vi "DWF Dig Query Line Configuration.vi"(0 "Instrument Handle In":u32, 11 "Error In":errorcluster caption="Error In (no error)") -> (4 "Instrument Handle Out":u32, 6 "Tristate Lines":string caption="Trigger Pattern", 8 "Static Lines":string caption="Trigger Pattern", 15 "Error Out":errorcluster)   [LabVIEW 2015, in "DigilentWF.lvlib"]
doc: "Indicates the current line configurations. <B>Tristate Lines</B>, <B>Static Lines</B>, and <B>Export Lines</B> contain comma-separated range and/or colon-delimited lists of all lines specified in Dig Initialize"
uses:
  <vilib>/DigilentWF/DigilentWF.lvlib
  dwf.dll
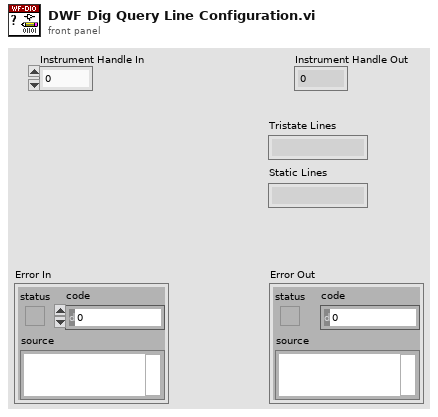
[diagram p1: front panel]
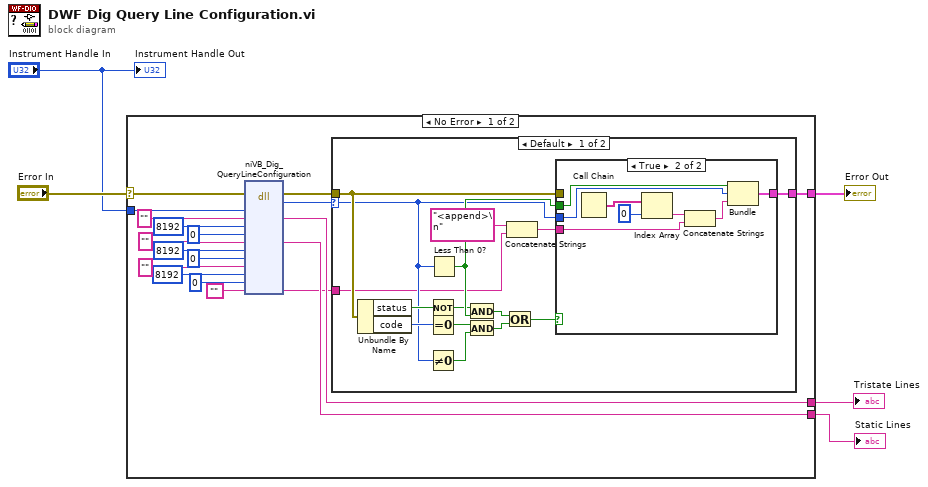
[diagram p0: block diagram]
diagram:
  n1 = case "outter_case" shown="No Error" "Error In" {
    selector: "Error In" -> [w19 w49]
    tunnel: [w23 w49] -> w4
    tunnel: "Instrument Handle In" -> [w10 _]
    tunnel: [w9 _] -> w2
    tunnel: [w8 _] -> w1
    frame No Error {
      n2 = dll-call lib="dwf.*" fn="niVB_Dig_QueryLineConfiguration"(error in=w19, "instrumentHandle"=w10, "tristateLines"="", "tristateLinesSize"=8192, "tristateLinesSizeOut"=0, "staticLines"="", "staticLinesSize"=8192, "staticLinesSizeOut"=0, "exportLines"="", "exportLinesSize"=8192, "exportLinesSizeOut"=0, "szError"="") -> (error out=w18:errorcluster, "return type"=w11:u32, "tristateLines"=w9:string, "staticLines"=w8:string, "szError"=w6:string)  [unwired: 10 in, 1 out]
      n3 = case "inner_case" shown="Default" w11 {
        selector: w11 -> [w28 _]
        tunnel: w18 -> [w29 w48]
        tunnel: [w25 w48] -> w23
        tunnel: w6 -> [w24 _]
        frame Default {
          n4 = Unbundle By Name(w29) -> ("status"=w33:bool, "code"=w37:i32)
          n5 = Not(x=w33) -> (.not. x?=w36:bool)
          n6 = Equal To 0?(x=w37) -> (x = 0?=w32:bool)
          n7 = Not Equal To 0?(x=w28) -> (x != 0?=w35:bool)
          n8 = Less Than 0?(x=w28) -> (x < 0?=w38:bool)
          n9 = And(x=w36, y=w38) -> (x .and. y?=w34:bool)
          n10 = And(x=w32, y=w35) -> (x .and. y?=w31:bool)
          n11 = Or(x=w34, y=w31) -> (x .or. y?=w30:bool)
          n12 = Concatenate Strings("<append>\n" ("string"), w24) -> (w27:string)
          n13 = case shown="True" w30 {
            tunnel: [w39 w46] -> w25
            tunnel: w28 -> [_ w45]
            tunnel: w38 -> [_ w44]
            tunnel: w29 -> [w39 _]
            tunnel: w27 -> [_ w40]
            frame False {
            }
            frame True {
              n14 = Call Chain() -> (call chain=w43:string[])
              n15 = Index Array(array=w43, index=0) -> (element=w42:string)
              n16 = Concatenate Strings(w42, w40) -> (w47:string)
              n17 = Bundle(w44, "return type"=w45, w47) -> (w46:cluster{bool, "return type":u32, string})  [unwired: 1 out]
            }
          }
        }
        frame 0 {
        }
      }
    }
    frame Error {
    }
  }
  "Error Out" <- w4
  "Tristate Lines" <- w2
  "Static Lines" <- w1
  "Instrument Handle Out" <- "Instrument Handle In"
